vi "Teleop.vi"(10 "Match Info":T1={"Autonomous Elapsed Seconds"=0.0, "TeleOp Elapsed Seconds"=0.0, "Disabled Elapsed Seconds"=0.0, "Visited Autonomous"=FALSE, "Visited TeleOp"=FALSE, "Visited Disabled"=FALSE, "Autonomous Settings"={"Autonomous Style"=enum."Independent", "VI Refnum"=refnum}}, 11 "Call Context":T2) -> ()   [LabVIEW 2018]
doc: "This VI is called for each TeleOp packet received from the DS where the robot is not disabled. It is often used to read from the joysticks and update I/O or to update setpoints for timed control loops. It should complete and return within 20 milliseconds or it may miss DS packets."
uses:
  <vilib>/Rock Robotics/WPI/DriverStation/WPI_DriverStationDerivedRobotMode.ctl
  <vilib>/Rock Robotics/WPI/DriverStation/WPI_DriverStationMatch Info.ctl
  RobotGlobal.vi
  Classes/Drive/Drive.lvclass
  Classes/Pnematics control/Pneumatics.lvclass
  Classes/Joysticks/Joysticks.lvclass
  Classes/Elevator/Elevator.lvclass
  Classes/Hatch/Hatch.lvclass
  Classes/Cargo/Cargo.lvclass
  Classes/Pnematics control/Solenoids/Solenoids.lvclass
  Classes/Vision/Vision.lvclass
panel:
  in  "calibrateElevator":bool
  out "error out":errorcluster
  in  "error in (no error)":errorcluster
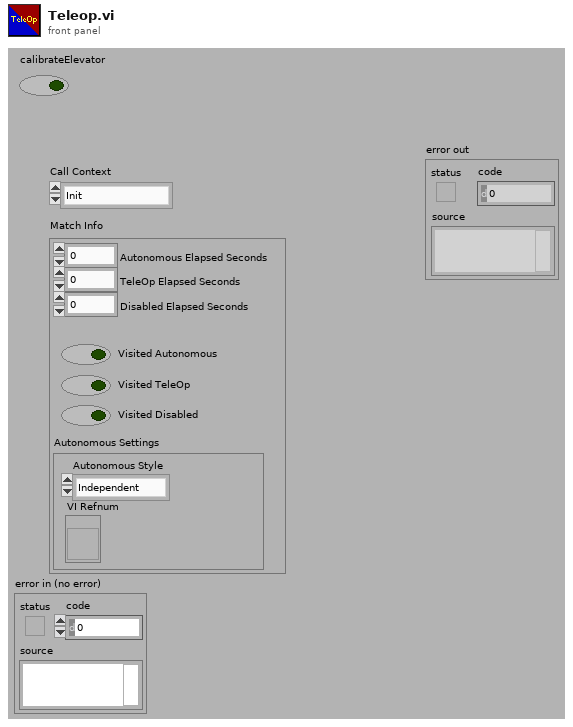
[diagram p1: front panel]
types:
  T1 = typedef "WPI_DriverStationMatch Info.ctl" = cluster{"Autonomous Elapsed Seconds":dbl, "TeleOp Elapsed Seconds":dbl, "Disabled Elapsed Seconds":dbl, "Visited Autonomous":bool, "Visited TeleOp":bool, "Visited Disabled":bool, "Autonomous Settings":cluster{"Autonomous Style":enum16{"Iterative", "Independent"}, "VI Refnum":refnum<vi>}}
  T2 = typedef "WPI_DriverStationDerivedRobotMode.ctl" = enum16{"Init", "Execute", "Stop"}
  T3 = typedef "RobotObjects.ctl" = cluster{"Drive.lvclass":refnum<class "Drive.lvclass">, "Pneumatics.lvclass":refnum<class "Pneumatics.lvclass">, "Vision.lvclass":refnum<class "Vision.lvclass">, "Joysticks.lvclass":refnum<class "Joysticks.lvclass">, "Elevator.lvclass":refnum<class "Elevator.lvclass">, "Hatch.lvclass":refnum<class "Hatch.lvclass">, "Cargo.lvclass":refnum<class "Cargo.lvclass">}
  T4 = typedef "Joysticks.lvlib/Joysticks.lvclass/JoystickData.ctl" = cluster{"X Axis":dbl, "Y Axis":dbl, "Drivetrain Shifter (Hold)":bool, "Beak (Toggle)":bool, "Cargo In (Hold)":bool, "Cargo Out (Hold)":bool, "Switch to hatch(toggle)":bool, "Switch to cargo(toggle)":bool, "Elevator Up (Toggle)":bool, "Elevator Down (Toggle)":bool, "AutoForward (Hold)":bool, "Climb(toggle)":bool, "Disengage Climb(toggle)":bool, "AutoTurn(hold)":bool, "CamMode(Two Driver only)":bool, "AltPipeline":bool}
  T5 = typedef "Elevator.lvlib/Elevator.lvclass/Elevator Position.ctl" = enum16{"CS, Cargo Ship Cargo", "C0, Cargo Ground", "C1, LV1 Cargo", "C2, LV2 Cargo", "C3, LV3 Cargo", "H0, LV1 Hatch", "H1, LV2 Hatch", "H2, LV3 Hatch"}
  T6 = typedef "Pneumatics control.lvlib/Pneumatics.lvclass/Solenoids.ctl" = cluster{"DriveShift":refnum<class "Solenoids.lvclass">, "ArmLock":refnum<class "Solenoids.lvclass">, "HatchArm":refnum<class "Solenoids.lvclass">, "HatchGrabber":refnum<class "Solenoids.lvclass">}
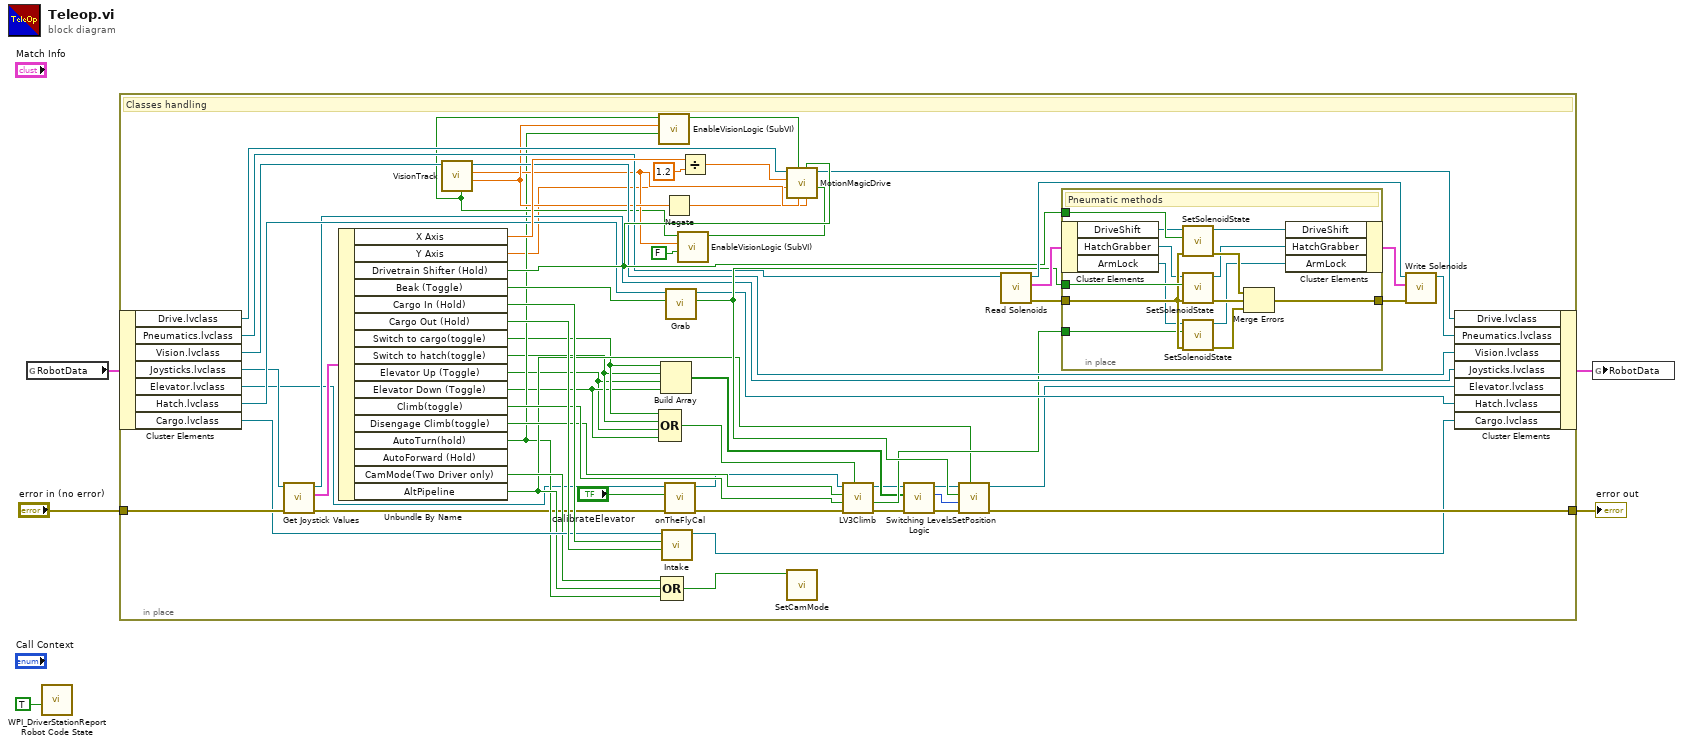
[diagram p0: block diagram]
diagram:
  n1 = global read "RobotGlobal.vi" "RobotData"() -> (w3:T3)
  n2 = call <vilib>:"WPI_DriverStationReport Robot Code State.vi"("TeleOp"=TRUE ("Autonomous")) -> ()  [unwired: 10 in, 1 out]
  n3 = in-place {
    in-place-border: "error in (no error)" -> [w50]
    in-place-border: [w49] -> w1
    # "Classes handling"
    n4 = in-place-cluster #1(w3) -> ("Drive.lvclass"=w60:refnum<class "Drive.lvclass">, "Pneumatics.lvclass"=w42:refnum<class "Pneumatics.lvclass">, "Vision.lvclass"=w40:refnum<class "Vision.lvclass">, "Joysticks.lvclass"=w38:refnum<class "Joysticks.lvclass">, "Elevator.lvclass"=w15:refnum<class "Elevator.lvclass">, "Hatch.lvclass"=w44:refnum<class "Hatch.lvclass">, "Cargo.lvclass"=w46:refnum<class "Cargo.lvclass">)
    n5 = call-dynamic "Get Joystick Values.vi"("error in (no error)"=w50, "Joysticks in"=w38) -> ("error out"=w13:errorcluster, "Joystick Data"=w51:T4, "Joysticks out"=w37:refnum<class "Joysticks.lvclass">)  [unwired: 7 in]
    n6 = Unbundle By Name(w51) -> ("X Axis"=w58:dbl, "Y Axis"=w16:dbl, "Drivetrain Shifter (Hold)"=w57:bool, "Beak (Toggle)"=w56:bool, "Cargo In (Hold)"=w55:bool, "Cargo Out (Hold)"=w54:bool, "Switch to cargo(toggle)"=w20:bool, "Switch to hatch(toggle)"=w19:bool, "Elevator Up (Toggle)"=w17:bool, "Elevator Down (Toggle)"=w18:bool, "Climb(toggle)"=w53:bool, "Disengage Climb(toggle)"=w52:bool, "AutoTurn(hold)"=w22:bool, "CamMode(Two Driver only)"=w25:bool, "AltPipeline"=w23:bool)  [unwired: 1 out]
    n7 = call "VisionTrack.vi"("Vision in"=w40) -> ("VerticalOffset(degrees)"=w32:dbl, "HorizontalOffset(degrees)"=w30:dbl, "Vision out"=w39:refnum<class "Vision.lvclass">, "Target?"=w28:bool)  [unwired: 5 in, 2 out]
    n8 = call "EnableVisionLogic (SubVI).vi"("Activate?(hold)"=w22, "Offset(degrees)"=w32, "Target?"=w28) -> ("Enable?"=w31:bool)  [unwired: 8 in]
    n9 = Compound Arithmetic op=OR(w20, w19, w17, w18) -> (w59:bool)
    n10 = Build Array(w20, w19, w17, w18) -> (w21:bool[])
    n11 = Compound Arithmetic op=OR(w25, w23, w22) -> (w24:bool)
    n12 = call-dynamic "Intake.vi"("Out"=w54, "In"=w55, "Cargo in"=w46) -> ("Cargo out"=w45:refnum<class "Cargo.lvclass">)  [unwired: 7 in, 1 out]
    n13 = Negate(x=w32) -> (-x=w27:dbl)
    n14 = call-dynamic "onTheFlyCal.vi"("error in (no error)"=w13, "calibrateElevator"="calibrateElevator", "Elevator in"=w15) -> ("error out"=w12:errorcluster, "Elevator out"=w14:refnum<class "Elevator.lvclass">)  [unwired: 7 in]
    n15 = call-dynamic "Grab.vi"("Grab Toggle?"=w56, "Hatch in"=w44) -> ("Solenoid On?"=w48:bool, "Hatch out"=w43:refnum<class "Hatch.lvclass">)  [unwired: 7 in, 1 out]
    n16 = call "EnableVisionLogic (SubVI).vi"("Activate?(hold)"=FALSE, "Offset(degrees)"=w30, "Target?"=w28) -> ("Enable?"=w29:bool)  [unwired: 8 in]
    n17 = Divide(x=w58, y=1.2) -> (x/y=w34:dbl)
    n18 = call-dynamic "MotionMagicDrive.vi"("Enable Vision Y"=w29, "X offset"=w27, "High gear?"=w57, "Y offset"=w30, "Enable Vision X"=w31, "Y Axis"=w16, "X Axis"=w34, "Drive in"=w60) -> ("Drive out"=w47:refnum<class "Drive.lvclass">)  [unwired: 2 in, 1 out]
    n19 = call "SetCamMode.vi"("Vision Processing?"=w24) -> ()  [unwired: 11 in]
    n20 = call-dynamic "LV3Climb.vi"("Deactivate?"=w59, "error in (no error)"=w12, "Activate?"=w53, "Redeploy?"=w52, "Elevator in"=w14) -> ("error out"=w11:errorcluster, "activate wrist lock"=w35:bool, "Elevator out"=w10:refnum<class "Elevator.lvclass">)  [unwired: 4 in]
    n21 = call "Switching Levels Logic.vi"("error in (no error)"=w11, "buttons"=w21, "Elevator in"=w10) -> ("error out"=w9:errorcluster, "Cargo/Hatch"=w8:T5, "Elevator out"=w7:refnum<class "Elevator.lvclass">)  [unwired: 6 in]
    n22 = call-dynamic "SetPosition.vi"("AltPipe?"=w23, "error in (no error)"=w9, "Position"=w8, "Hatch Grabbed?"=w48, "Elevator in"=w7) -> ("error out"=w49:errorcluster, "Elevator out"=w36:refnum<class "Elevator.lvclass">)  [unwired: 5 in]
    n23 = call-dynamic "Read Solenoids.vi"("Pneumatics in"=w42) -> ("error out"=w63:errorcluster, "Solenoids"=w62:T6, "Pneumatics out"=w61:refnum<class "Pneumatics.lvclass">)  [unwired: 8 in]
    n24 = in-place {
      in-place-border: w57 -> [w78]
      in-place-border: w63 -> [w72]
      in-place-border: [w76] -> w65
      in-place-border: w48 -> [w74]
      in-place-border: w35 -> [w71]
      # "Pneumatic methods"
      n25 = in-place-cluster #2(w62) -> ("DriveShift"=w70:refnum<class "Solenoids.lvclass">, "HatchGrabber"=w69:refnum<class "Solenoids.lvclass">, "ArmLock"=w68:refnum<class "Solenoids.lvclass">)
      n26 = call-dynamic "SetSolenoidState.vi"("error in (no error)"=w72, "Solenoid On?"=w78, "Solenoids in"=w70) -> ("error out"=w77:errorcluster, "Solenoids out"=w79:refnum<class "Solenoids.lvclass">)  [unwired: 7 in]
      n27 = call-dynamic "SetSolenoidState.vi"("error in (no error)"=w72, "Solenoid On?"=w74, "Solenoids in"=w69) -> ("error out"=w75:errorcluster, "Solenoids out"=w67:refnum<class "Solenoids.lvclass">)  [unwired: 7 in]
      n28 = call-dynamic "SetSolenoidState.vi"("error in (no error)"=w72, "Solenoid On?"=w71, "Solenoids in"=w68) -> ("error out"=w73:errorcluster, "Solenoids out"=w66:refnum<class "Solenoids.lvclass">)  [unwired: 7 in]
      n29 = Merge Errors(w77, w75, w73) -> (w76:errorcluster)
      n30 = in-place-cluster #2("DriveShift"=w79, "HatchGrabber"=w67, "ArmLock"=w66) -> (w64:T6)
    }
    n31 = call-dynamic "Write Solenoids.vi"("error in (no error)"=w65, "Solenoids"=w64, "Pneumatics in"=w61) -> ("Pneumatics out"=w41:refnum<class "Pneumatics.lvclass">)  [unwired: 7 in, 1 out]
    n32 = in-place-cluster #1("Drive.lvclass"=w47, "Pneumatics.lvclass"=w41, "Vision.lvclass"=w39, "Joysticks.lvclass"=w37, "Elevator.lvclass"=w36, "Hatch.lvclass"=w43, "Cargo.lvclass"=w45) -> (w4:T3)
  }
  "error out" <- w1
  n33 = global write "RobotGlobal.vi" "RobotData"(w4) -> ()
